vi "XYStage.KIM101.DVRtoRef.vi"(10 "Ref":T1) -> (2 "Ref":u32 format="%08x")   [LabVIEW 2017, in "XYStage.KIM101.lvclass"]
doc: "JKI State Machine Objects (SMO) 1.0.0.5\nJKI - JKI\nCopyright (c) 2016, JKI"
uses:
  XYStage.KIM101.lvclass
  Typedefs/PrivateData--Ref.ctl
  Typedefs/PrivateData--Cluster.ctl
  Typedefs/Resource--Cluster.ctl
  D:/upwork/Laser Measurement Tool/Laser/project/data/Thorlabs.MotionControl.Controls.dll
  data/Thorlabs.MotionControl.Controls.dll
  D:/upwork/Laser Measurement Tool/Laser/project/data/Thorlabs.MotionControl.KCube.InertialMotorCLI.dll
  data/Thorlabs.MotionControl.KCube.InertialMotorCLI.dll
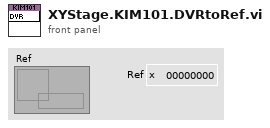
[diagram p1: front panel]
types:
  T1 = typedef "XYStage.KIM101.lvclass/PrivateData--Ref.ctl" = refnum<data-value>
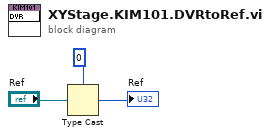
[diagram p0: block diagram]
diagram:
  n1 = Type Cast(type=u32 0 ("Ref"), x="Ref") -> (*(type *) &x=→"Ref":u32)
